vi "ChassisControlLoop.vi"   [LabVIEW 2014, in "ChassisLib.lvlib"]
uses:
  ChassisLib.lvlib
  ChassisRefs.ctl
  <vilib>/Rock Robotics/WPI/RobotDrive/WPI_RobotDriveGetSetRefNum.vi
  <vilib>/Rock Robotics/Network Tables/SD Write Number.vi
types:
  T1 = typedef "ChassisLib.lvlib/ChassisRefs.ctl" = enum16{"RobotDrive", "Compressor", "DriveEncoderLeft", "DriveEncoderRight", "RioAccel"}
  T2 = typedef "WPI_EncoderDevRef.ctl" = cluster{"DevStatus":errorcluster, "EncoderIndex":T3, "CounterIndex":T4, "DistancePerCount":dbl, "Decoding Type":T5}
  T3 = typedef "FPGA_EncoderIdx.ctl" = enum8{"Enc 0", "Enc 1", "Enc 2", "Enc 3", "Enc 4", "Enc 5", "Enc 6", "Enc 7", "Invalid"}
  T4 = typedef "FPGA_CounterCtrSystemIndex.ctl" = enum8{"Ctr 0", "Ctr 1", "Ctr 2", "Ctr 3", "Ctr 4", "Ctr 5", "Ctr 6", "Ctr 7", "Invalid"}
  T5 = typedef "WPI_EncoderType.ctl" = enum16{"1x", "2x", "4x"}
  T6 = typedef "WPI_RobotDriveDevRef.ctl" = cluster{"DevStatus":errorcluster, "Motors[]":T7[], "Square Inputs":bool, "Max Output":dbl}
  T7 = typedef "WPI_MotorControlDeviceRef.ctl" = cluster{"DeviceStatus":errorcluster, "Type":T8, "PWM":cluster{"Controller":T9, "PWM Channel":T10, "DeadBand":T11}, "CAN":cluster{"Device Number":u8, "Control Mode":T12, "Semaphore":T13, "Max Vout":dbl, "TalonSRX Control Mode":T14}, "Invert":bool, "TransformRef":T15, "InvTransformRef":T15}
  T8 = typedef "WPI_MotorControlType.ctl" = enum16{"PWM", "CAN", "CANTalonSRX"}
  T9 = typedef "FPGA_TypedefDigitalModule.ctl" = enum16{"Controller 1"}
  T10 = typedef "FPGA_DIOPWMChannel.ctl" = enum8{"PWM 0", "PWM 1", "PWM 2", "PWM 3", "PWM 4", "PWM 5", "PWM 6", "PWM 7", "PWM 8", "PWM 9", "PWM MXP 0", "PWM MXP 1", "PWM MXP 2", "PWM MXP 3", "PWM MXP 4", "PWM MXP 5", "PWM MXP 6", "PWM MXP 7", "PWM MXP 8", "PWM MXP 9", "Invalid"}
  T11 = typedef "WPI_PWMDeadband.ctl" = cluster{"Name":string, "maxPositivePwm":i32, "minPositivePwm":i32, "centerPwm":i32, "maxNegativePwm":i32, "minNegativePwm":i32, "angularRange":u16}
  T12 = typedef "WPI_CANJaguar_ControlMode.ctl" = enum8{"Percent VBus", "Current", "Speed", "Position", "Voltage"}
  T13 = typedef "Semaphore RefNum" = refnum<k1>
  T14 = typedef "WPI_CANTalonSRX_APIControlMode.ctl" = enum8{"Percent VBus", "Speed", "Position", "Slave", "Unchanged / Invalid"}
  T15 = typedef "WPI_PWMTransform_ConPane.ctl" = refnum<vi>
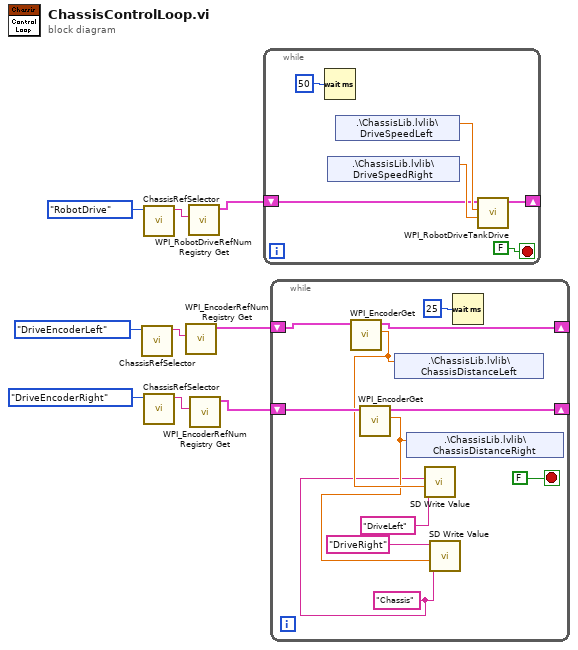
[diagram p0: block diagram]
diagram:
  n1 = call "ChassisRefSelector.vi"("Enum 2"=ChassisRefs."DriveEncoderLeft") -> ("String"=w4:string)  [unwired: 10 in]
  n2 = call "ChassisRefSelector.vi"("Enum 2"=ChassisRefs."RobotDrive") -> ("String"=w8:string)  [unwired: 10 in]
  n3 = call "ChassisRefSelector.vi"("Enum 2"=ChassisRefs."DriveEncoderRight") -> ("String"=w3:string)  [unwired: 10 in]
  n4 = call <vilib>:"WPI_EncoderRefNum Registry Get.vi"("refnum name"=w4) -> ("EncoderDevRef"=w1:T2)  [unwired: 9 in, 1 out]
  n5 = call <vilib>:"WPI_RobotDriveRefNum Registry Get.vi"("refnum name"=w8) -> ("RobotDriveDevRef"=w7:T6)  [unwired: 9 in, 1 out]
  n6 = call <vilib>:"WPI_EncoderRefNum Registry Get.vi"("refnum name"=w3) -> ("EncoderDevRef"=w2:T2)  [unwired: 9 in, 1 out]
  n7 = while {
    shift-right: [w10] -> _
    shift-left: w7 -> [w11]
    stop <- FALSE stop-if-true
    n8 = Wait (ms)(milliseconds to wait=u32 50) -> ()  [unwired: 1 out]
    n9 = shared-variable ".\\ChassisLib.lvlib\\DriveSpeedRight"() -> (w13:dbl)  [unwired: 1 in, 1 out]
    n10 = shared-variable ".\\ChassisLib.lvlib\\DriveSpeedLeft"() -> (w12:dbl)  [unwired: 1 in, 1 out]
    n11 = call <vilib>:"WPI_RobotDriveTankDrive.vi"("Right axis value"=w13, "Left axis value"=w12, "RobotDriveDevRef"=w11) -> ("RobotDriveDevRef"=w10:T6)  [unwired: 6 in, 2 out]
  }
  n12 = while {
    shift-right: [w25] -> _
    shift-left: w2 -> [w26]
    shift-right: [w23] -> _
    shift-left: w1 -> [w24]
    stop <- FALSE stop-if-true
    w16 = "Chassis" ("Table Prefix")
    n13 = call <vilib>:"WPI_EncoderGet.vi"("EncoderDevRef"=w24) -> ("Distance"=w18:dbl, "EncoderDevRef"=w23:T2)  [unwired: 5 in, 4 out]
    n14 = call <vilib>:"WPI_EncoderGet.vi"("EncoderDevRef"=w26) -> ("Distance"=w17:dbl, "EncoderDevRef"=w25:T2)  [unwired: 5 in, 4 out]
    n15 = shared-variable ".\\ChassisLib.lvlib\\ChassisDistanceLeft"(w18) -> ()  [unwired: 1 in, 1 out]
    n16 = shared-variable ".\\ChassisLib.lvlib\\ChassisDistanceRight"(w17) -> ()  [unwired: 1 in, 1 out]
    n17 = call-poly <vilib>:"SD Write Value.vi"("Numeric"=w18, "Table Prefix"=w16, "Name"="DriveLeft") -> ()  [unwired: 7 in, 2 out]
    n18 = call-poly <vilib>:"SD Write Value.vi"("Numeric"=w17, "Table Prefix"=w16, "Name"="DriveRight") -> ()  [unwired: 7 in, 2 out]
    n19 = Wait (ms)(milliseconds to wait=u32 25) -> ()  [unwired: 1 out]
  }
